vi "fetch_translation_request.vi"(8 "error in (no error)":errorcluster, 11 "GenericStage in":refnum<class "GenericStage.lvclass">) -> (0 "error out":errorcluster, 3 "GenericStage out":refnum<class "GenericStage.lvclass">)   [LabVIEW 2010, in "GenericStage.lvclass"]
uses:
  GenericStage.lvclass
  translation_request.ctl
  translation_mode_enum.ctl
  common/classes/SpaceVector/SpaceVector/SpaceVector.lvclass
  class_data.vi
  common/classes/ErrorController/ErrorController/class_data.vi
  common/classes/ErrorController/ErrorController/ErrorController.lvclass
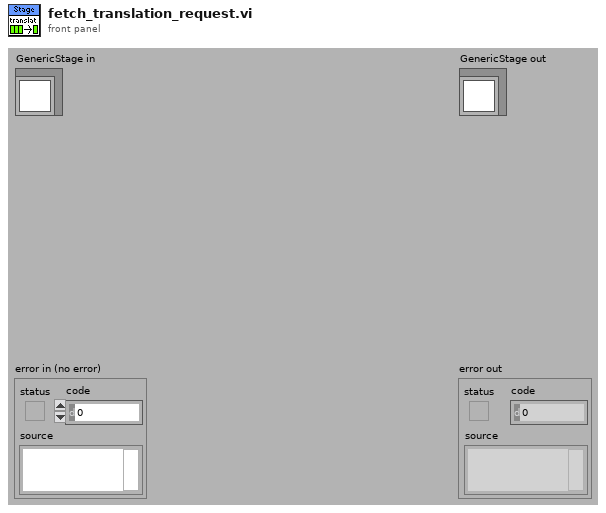
[diagram p1: front panel]
types:
  T1 = typedef "GenericStage.lvclass/translation_request.ctl" = cluster{"translation mode":T2, "translation vector":refnum<class "SpaceVector.lvclass">}
  T2 = typedef "GenericStage.lvclass/translation_mode_enum.ctl" = enum16{"DON'T MOVE", "relative", "absolute"}
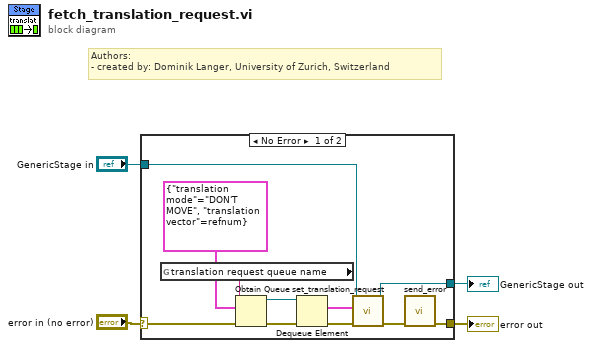
[diagram p0: block diagram]
diagram:
  # "Authors: \n- created by: Dominik Langer, University of Zurich, Switzerland"
  n1 = case shown="No Error" "error in (no error)" {
    selector: "error in (no error)" -> [w13 w17]
    tunnel: [w5 w17] -> w3
    tunnel: [w7 w16] -> w1
    tunnel: "GenericStage in" -> [w8 w16]
    frame No Error {
      n2 = global read "class_data.vi" "translation request queue name"() -> (w15:string)
      n3 = Obtain Queue(name (unnamed)=w15, element data type=T1 {"translation mode"=enum."DON'T MOVE", "translation vector"=refnum} ("translation request"), error in (no error)=w13) -> (queue out=w11:refnum<queue>, error out=w14:errorcluster)  [unwired: 2 in, 1 out]
      n4 = Dequeue Element(queue=w11, error in (no error)=w14) -> (element=w9:T1, error out=w10:errorcluster)  [unwired: 3 out]
      n5 = call-dynamic "set_translation_request.vi"("error in (no error)"=w10, "translation request"=w9, "GenericStage.lvclass in"=w8) -> ("error out"=w6:errorcluster, "GenericStage.lvclass out"=w7:refnum<class "GenericStage.lvclass">)  [unwired: 7 out]
      n6 = call "send_error.vi"("error in (no error)"=w6) -> ("error out"=w5:errorcluster)  [unwired: 10 in]
    }
    frame Error {
    }
  }
  "error out" <- w3
  "GenericStage out" <- w1
